vi "Util_Progress Close Progress Popup.vi"(8 "error in (no error)":errorcluster) -> (0 "error out":errorcluster)   [LabVIEW 2016]
panel:
  out "appended path":path
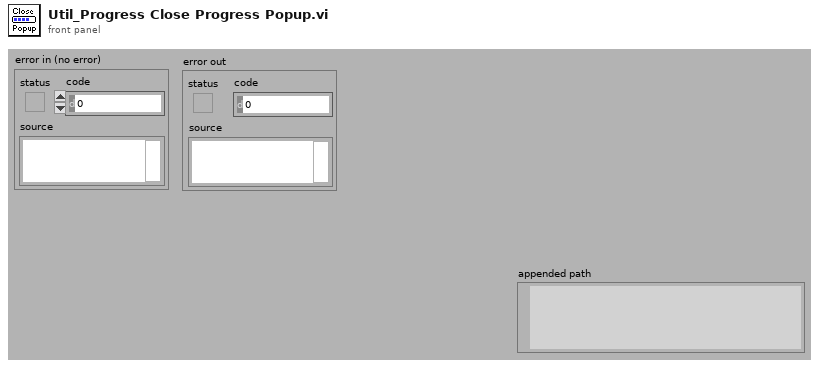
[diagram p1: front panel]
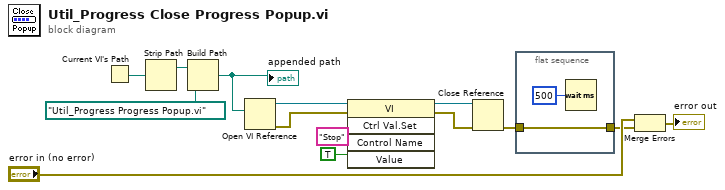
[diagram p0: block diagram]
diagram:
  n1 = Current VI's Path() -> (path=w14:path)
  n2 = Strip Path(path=w14) -> (stripped path=w13:path)  [unwired: 1 out]
  n3 = Build Path(base path=w13, name or relative path=path "Util_Progress Progress Popup.vi" ("vi path")) -> (appended path=w11:path)
  "appended path" <- w11
  n4 = Open VI Reference(vi path=w11) -> (vi reference=w6:refnum<vi>, error out=w4:errorcluster)  [unwired: 1 in, 4 out]
  n5 = invoke class="VI" method="Ctrl Val.Set"(reference=w6, error in=w4, "Control Name"="Stop", "Value"=TRUE) -> (reference out=w9:refnum<vi>, error out=w10:errorcluster)  [unwired: 1 in, 3 out]
  n6 = Close Reference(reference=w9, error in (no error)=w10) -> (error out=w5:errorcluster)
  n7 = flat-sequence {
    tunnel: w5 -> [w16]
    tunnel: [w16] -> w1
    frame #0 {
      n8 = Wait (ms)(milliseconds to wait=u32 500) -> ()  [unwired: 1 out]
    }
  }
  n9 = Merge Errors("error in (no error)", w1) -> (→"error out":errorcluster)
